vi "Robot Properties.vi"() -> ()   [LabVIEW 2018]
panel:
  in  "Lidar Offset (mm)":dbl=100.0
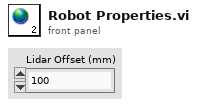
[diagram p1: front panel]
diagram:
